vi "Message.vi"(8 "error in (no error)":errorcluster, 11 "Node Ptr":T2 format="%.0x") -> (0 "error out":errorcluster)   [LabVIEW 2019, in "Instrument Addon System Explorer.lvlib"]
uses:
  Instrument Addon System Explorer.lvlib
  <vilib>/NI VeriStand/Custom Device API/Custom Device Item Ref.ctl
  Addon Shared/Types/Message Generation Type.ctl
  Addon Shared/Types/FG Control.ctl
  Addon Shared/SubVIs/Constants.vi
  <vilib>/NI VeriStand/Custom Device API/NI VeriStand - Get Item Property.vi
  <vilib>/NI VeriStand/Custom Device API/Get Item Property (U32).vi
  <vilib>/NI VeriStand/Custom Device API/Get Item Property (Double).vi
  <vilib>/NI VeriStand/Custom Device API/Get Item Property (Boolean).vi
  <vilib>/NI VeriStand/Custom Device API/Get Item Property (String).vi
  <vilib>/NI VeriStand/Custom Device API/NI VeriStand - Set Item Property.vi
  <vilib>/NI VeriStand/Custom Device API/Set Item Property (U32).vi
  <vilib>/NI VeriStand/Custom Device API/Set Item Property (Double).vi
  <vilib>/NI VeriStand/Custom Device API/Set Item Property (Boolean).vi
  <vilib>/NI VeriStand/Custom Device API/Set Item Property (String).vi
  <vilib>/NI VeriStand/Custom Device API/Custom Device API.lvlib
  Addon Shared/Instrument Addon Shared.lvlib
panel:
  in  "Type":string(combo)
  in  "Include Protection":bool caption="Include Protection?"
  in  "Period":dbl=1.0 caption="Period (sec)" format="%#_p"
  in  "Generation Type":T1
  in  "Header 2":cluster{"Section Name":string}={"Section Name"="Generation Settings"}
  in  "SHDocVw.IWebBrowser":refnum<k7>(container)
  in  "Header":cluster{"Section Name":string}={"Section Name"="Message Settings"}
  in  "Description":string
  in  "Name":string
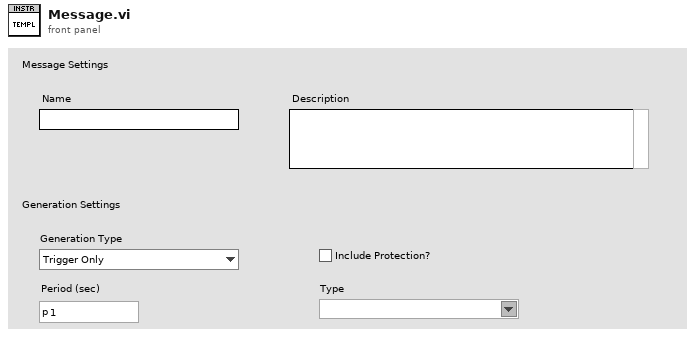
[diagram p1: front panel]
types:
  T1 = typedef "Instrument Addon Shared.lvlib/Message Generation Type.ctl" = enum16{"Trigger Only", "Periodic & Trigger", "Value Change & Trigger"}
  T2 = typedef "Custom Device API.lvlib/Custom Device Item Ref.ctl" = u64
  T3 = typedef "Instrument Addon Shared.lvlib/FG Control.ctl" = enum16{"Get", "Set"}
  T4 = typedef "Instrument Addon Shared.lvlib/Message Parameters.ctl" = cluster{"Generation Type":T1, "Period":dbl, "Include Protection":bool, "Type":string}
  T5 = typedef "Custom Device API.lvlib/Custom Device Item Info.ctl" = cluster{"Name":string, "Is Channel":bool, "GUID":string, "Is Waveform":bool}
  T6 = typedef "Custom Device API.lvlib/Custom Device Commands.ctl" = enum16{"Default", "Item renamed", "Shutdown", "Dynamic button pressed"}
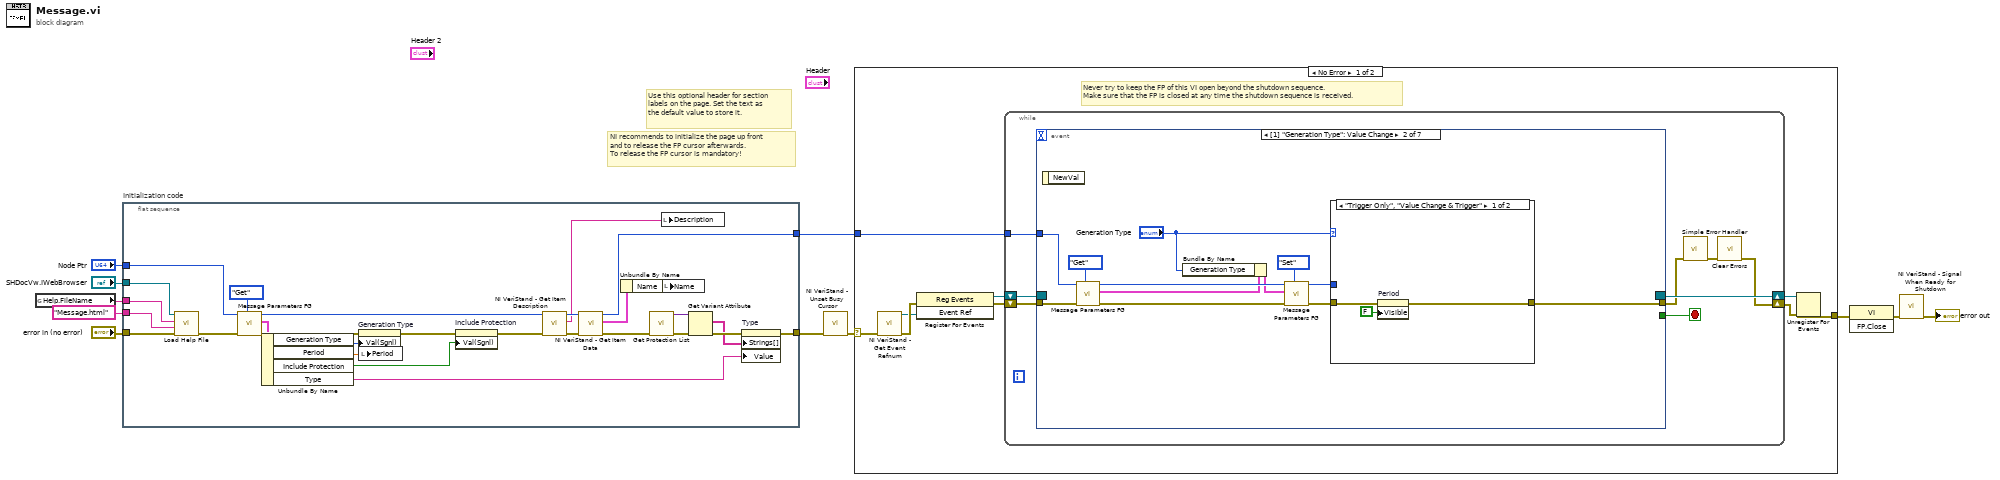
[diagram p0: block diagram]
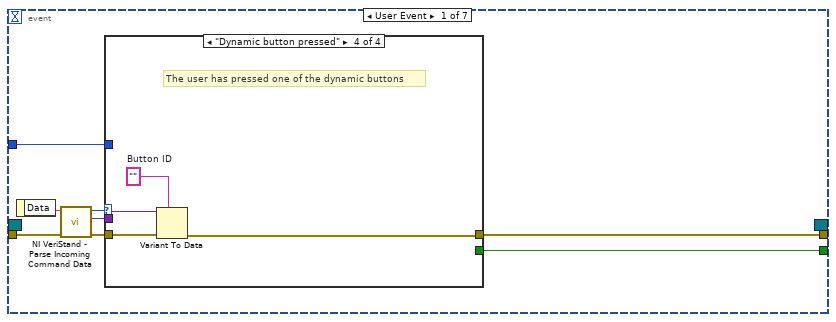
[diagram p2: hidden frame]
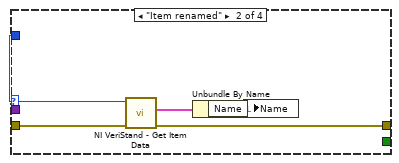
[diagram p4: hidden frame]
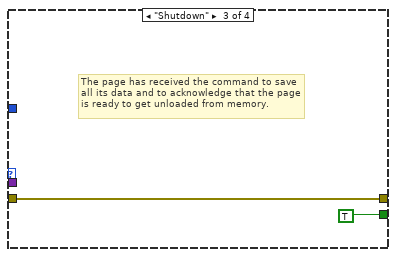
[diagram p5: hidden frame]
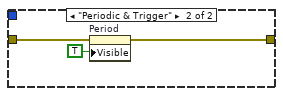
[diagram p6: hidden frame]
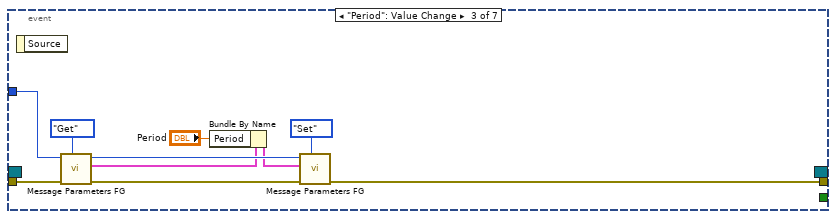
[diagram p7: hidden frame]
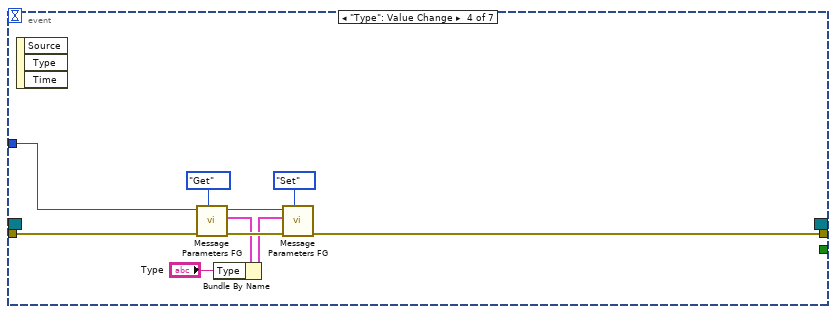
[diagram p8: hidden frame]
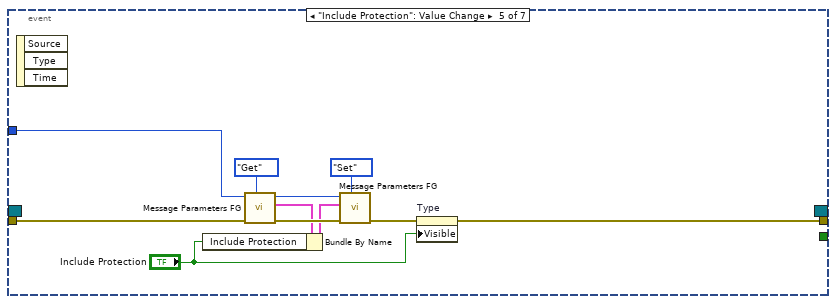
[diagram p9: hidden frame]
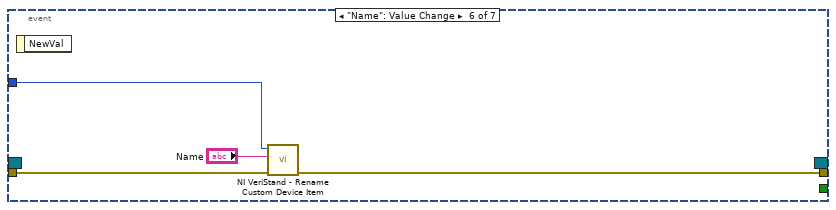
[diagram p10: hidden frame]
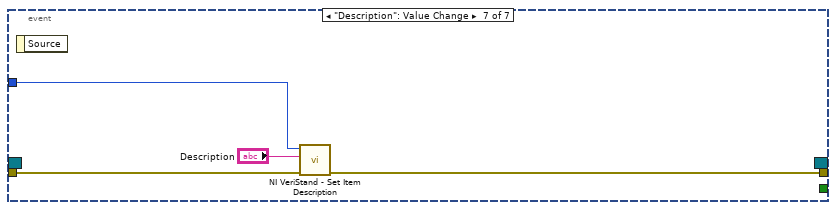
[diagram p11: hidden frame]
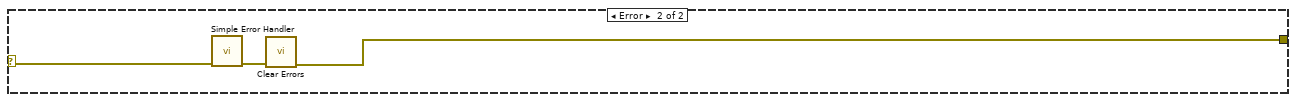
[diagram p12: hidden frame]
diagram:
  # "Use this optional header for section labels on the page. Set the text as the default value to store it."
  # "NI recommends to initialize the page up front\nand to release the FP cursor afterwards.\nTo release the FP cursor is mandatory!"
  n1 = global read "Constants.vi" "Help.FileName"() -> (w1:string)
  n2 = flat-sequence "Initialization code" {
    tunnel: "error in (no error)" -> [w33]
    tunnel: "Node Ptr" -> [w27]
    tunnel: [w13] -> w7
    tunnel: [w39] -> w4
    tunnel: "SHDocVw.IWebBrowser" -> [w32]
    tunnel: w1 -> [w31]
    tunnel: "Message.html" ("HTML File") -> [w30]
    frame #0 {
      n3 = call "Load Help File.vi"("error in (no error)"=w33, "HTML File"=w30, "Main CHM File"=w31, "SHDocVw.IWebBrowser2"=w32) -> ("error out"=w28:errorcluster)  [unwired: 7 in]
      n4 = call "Message Parameters FG.vi"("Action"=FG_Control."Get", "error in (no error)"=w28, "Item Ref in"=w27) -> ("error out"=w25:errorcluster, "Message Settings out"=w24:T4, "Item Ref out"=w26:T2)  [unwired: 6 in]
      n5 = Unbundle By Name(w24) -> ("Generation Type"=w23:T1, "Period"=w22:dbl, "Include Protection"=w20:bool, "Type"=w12:string)
      n6 = property on="Generation Type" class="Enum (strict)"(error in=w25, "Val(Sgnl)"=w23) -> (error out=w21:errorcluster)  [unwired: 1 in, 1 out]
      n7 = local write "Period"(w22) -> ()
      n8 = property on="Include Protection" class="Bool (strict)"(error in=w21, "Val(Sgnl)"=w20) -> (error out=w15:errorcluster)  [unwired: 1 in, 1 out]
      n9 = call <vilib>:"NI VeriStand - Get Item Description.vi"("error in (no error)"=w15, "Item Ref in"=w26) -> ("error out"=w36:errorcluster, "Description"=w37:string, "Item Ref out"=w38:T2)  [unwired: 7 out]
      n10 = call <vilib>:"NI VeriStand - Get Item Data.vi"("error in (no error)"=w36, "Item Ref in"=w38) -> ("error out"=w14:errorcluster, "Item Info"=w35:T5, "Item Ref out"=w39:T2)  [unwired: 7 out]
      n11 = Unbundle By Name(w35) -> ("Name"=w34:string)
      n12 = call "Get Protection List.vi"("error in (no error)"=w14) -> ("error out"=w19:errorcluster, "Class Lookup"=w17:variant)  [unwired: 9 in]
      n13 = local write "Description"(w37) -> ()
      n14 = local write "Name"(w34) -> ()
      n15 = Get Variant Attribute(Variant=w17, error in=w19) -> (names=w16:string[], error out=w18:errorcluster)  [unwired: 2 in, 2 out]
      n16 = property on="Type" class="CmbBox"(error in=w18, "Strings[]"=w16, "Value"=w12) -> (error out=w13:errorcluster)  [unwired: 1 in, 1 out]
    }
  }
  n17 = call <vilib>:"NI VeriStand - Unset Busy Cursor.vi"("error in (no error)"=w7) -> ("error out"=w6:errorcluster)  [unwired: 10 out]
  n18 = case shown="No Error" w6 {
    selector: w6 -> [w40 w136]
    tunnel: [w45 w134] -> w11
    tunnel: w4 -> [w41 _]
    frame No Error {
      # "Never try to keep the FP of this VI open beyond the shutdown sequence.\nMake sure that the FP is closed at any time the shutdown sequence is received."
      n19 = call <vilib>:"NI VeriStand - Get Event Refnum.vi"("error in (no error)"=w40) -> ("error out"=w48:errorcluster, "Event Ref"=w44:refnum<user-event>)  [unwired: 9 out]
      n20 = register-events(error in=w48, w44) -> (reference out=w42:refnum<event-registration>, error out=w43:errorcluster)  [unwired: 1 in]
      n21 = while {
        tunnel: w41 -> [w52]
        shift-right: [w49] -> w46
        shift-left: w43 -> [w55]
        shift-right: [w56] -> w47
        shift-left: w42 -> [w54]
        stop <- w53 stop-if-true
        n22 = event shown="[1] \"Generation Type\": Value Change" {
          selector: w54 -> [_ _ _ _ _ _ _]
          dyn-events: [_ _ _ _ _ _ _] -> w56
          timeout: _ -> [_ _ _ _ _ _ _]
          tunnel: w55 -> [w64 w88 w104 w114 w125 w129 w132]
          tunnel: [w60 _ _ _ _ _ _] -> w53
          tunnel: [w59 w79 w96 w106 w115 w128 w131] -> w51
          tunnel: w52 -> [w58 w87 w103 w113 w124 w127 w133]
          event User Event {
            n23 = event-data() -> ("Data"=w63:string)  [unwired: 1 out]
            n24 = call <vilib>:"NI VeriStand - Parse Incoming Command Data.vi"("error in (no error)"=w64, "Incoming data"=w63) -> ("error out"=w62:errorcluster, "Outgoing data"=w57:variant, "Action"=w61:T6)  [unwired: 7 out]
            n25 = case shown="\"Dynamic button pressed\"" w61 {
              tunnel: w62 -> [w65 w70 w71 w76]
              tunnel: [_ _ TRUE _] -> w60
              tunnel: [w65 w67 w71 w73] -> w59
              tunnel: w58 -> [_ w69 _ _]
              tunnel: w57 -> [_ _ _ w75]
              frame "Default", Default {
              }
              frame "Item renamed" {
                n26 = call <vilib>:"NI VeriStand - Get Item Data.vi"("error in (no error)"=w70, "Item Ref in"=w69) -> ("error out"=w67:errorcluster, "Item Info"=w68:T5)  [unwired: 8 out]
                n27 = Unbundle By Name(w68) -> ("Name"=w66:string)
                n28 = local write "Name"(w66) -> ()
              }
              frame "Shutdown" {
                # "The page has received the command to save all its data and to acknowledge that the page is ready to get unloaded from memory."
              }
              frame "Dynamic button pressed" {
                w74 = ""  # Button ID
                # "The user has pressed one of the dynamic buttons"
                n29 = Variant To Data(error in=w76, type=w74, Variant=w75) -> (error out=w73:errorcluster)  [unwired: 1 out]
              }
            }
          }
          event Value Change {
            n30 = event-data() -> ()  [unwired: 2 out]
            n31 = call "Message Parameters FG.vi"("Action"=FG_Control."Get", "error in (no error)"=w88, "Item Ref in"=w87) -> ("error out"=w86:errorcluster, "Message Settings out"=w83:T4, "Item Ref out"=w85:T2)  [unwired: 6 in]
            n32 = Bundle By Name(cluster=w83, "Generation Type"="Generation Type") -> (w82:T4)
            n33 = call "Message Parameters FG.vi"("Action"=FG_Control."Set", "error in (no error)"=w86, "Message Settings"=w82, "Item Ref in"=w85) -> ("error out"=w80:errorcluster, "Item Ref out"=w77:T2)  [unwired: 5 in, 1 out]
            n34 = case shown="\"Trigger Only\", \"Value Change & Trigger\"" "Generation Type" {
              tunnel: w80 -> [w90 w94]
              tunnel: [w89 w92] -> w79
              tunnel: w77 -> [_ _]
              frame "Trigger Only", "Value Change & Trigger" {
                n35 = property on="Period" class="DigNum (strict)"(error in=w90, "Visible"=FALSE) -> (error out=w89:errorcluster)  [unwired: 1 in, 1 out]
              }
              frame "Periodic & Trigger" {
                n36 = property on="Period" class="DigNum (strict)"(error in=w94, "Visible"=TRUE) -> (error out=w92:errorcluster)  [unwired: 1 in, 1 out]
              }
            }
          }
          event "Period": Value Change {
            n37 = event-data() -> ()  [unwired: 2 out]
            n38 = call "Message Parameters FG.vi"("Action"=FG_Control."Get", "error in (no error)"=w104, "Item Ref in"=w103) -> ("error out"=w102:errorcluster, "Message Settings out"=w99:T4, "Item Ref out"=w101:T2)  [unwired: 6 in]
            n39 = Bundle By Name(cluster=w99, "Period"="Period") -> (w98:T4)
            n40 = call "Message Parameters FG.vi"("Action"=FG_Control."Set", "error in (no error)"=w102, "Message Settings"=w98, "Item Ref in"=w101) -> ("error out"=w96:errorcluster)  [unwired: 5 in, 2 out]
          }
          event "Type": Value Change {
            n41 = event-data() -> ()  [unwired: 4 out]
            n42 = call "Message Parameters FG.vi"("Action"=FG_Control."Get", "error in (no error)"=w114, "Item Ref in"=w113) -> ("error out"=w112:errorcluster, "Message Settings out"=w109:T4, "Item Ref out"=w111:T2)  [unwired: 6 in]
            n43 = Bundle By Name(cluster=w109, "Type"="Type") -> (w108:T4)
            n44 = call "Message Parameters FG.vi"("Action"=FG_Control."Set", "error in (no error)"=w112, "Message Settings"=w108, "Item Ref in"=w111) -> ("error out"=w106:errorcluster)  [unwired: 5 in, 2 out]
          }
          event "Include Protection": Value Change {
            n45 = event-data() -> ()  [unwired: 4 out]
            n46 = call "Message Parameters FG.vi"("Action"=FG_Control."Get", "error in (no error)"=w125, "Item Ref in"=w124) -> ("error out"=w123:errorcluster, "Message Settings out"=w120:T4, "Item Ref out"=w122:T2)  [unwired: 6 in]
            n47 = Bundle By Name(cluster=w120, "Include Protection"="Include Protection") -> (w119:T4)
            n48 = call "Message Parameters FG.vi"("Action"=FG_Control."Set", "error in (no error)"=w123, "Message Settings"=w119, "Item Ref in"=w122) -> ("error out"=w116:errorcluster)  [unwired: 5 in, 2 out]
            n49 = property on="Type" class="CmbBox"(error in=w116, "Visible"="Include Protection") -> (error out=w115:errorcluster)  [unwired: 1 in, 1 out]
          }
          event "Name": Value Change {
            n50 = event-data() -> ()  [unwired: 2 out]
            n51 = call <vilib>:"NI VeriStand - Rename Custom Device Item.vi"("error in (no error)"=w129, "New Name"="Name", "Item Ref in"=w127) -> ("error out"=w128:errorcluster)  [unwired: 1 in, 7 out]
          }
          event "Description": Value Change {
            n52 = event-data() -> ()  [unwired: 2 out]
            n53 = call <vilib>:"NI VeriStand - Set Item Description.vi"("error in (no error)"=w132, "Description"="Description", "Item Ref in"=w133) -> ("error out"=w131:errorcluster)  [unwired: 8 out]
          }
        }
        n54 = call <vilib>:"Simple Error Handler.vi"("error in (no error)"=w51) -> ("error out"=w50:errorcluster)  [unwired: 1 in, 7 out]
        n55 = call <vilib>:"Clear Errors.vi"("error in (no error)"=w50) -> ("error out"=w49:errorcluster)  [unwired: 1 in, 5 out]
      }
      n56 = Unregister For Events(event registration refnum=w47, error in=w46) -> (error out=w45:errorcluster)
    }
    frame Error {
      n57 = call <vilib>:"Simple Error Handler.vi"("error in (no error)"=w136) -> ("error out"=w135:errorcluster)  [unwired: 1 in, 7 out]
      n58 = call <vilib>:"Clear Errors.vi"("error in (no error)"=w135) -> ("error out"=w134:errorcluster)  [unwired: 1 in, 5 out]
    }
  }
  n59 = invoke class="VI" method="FP.Close"(error in=w11) -> (error out=w10:errorcluster)  [unwired: 2 in, 2 out]
  n60 = call <vilib>:"NI VeriStand - Signal When Ready for Shutdown.vi"("error in (no error)"=w10) -> ("error out"=→"error out":errorcluster)  [unwired: 10 out]
